vi "Clear Received Replies.vi"(8 "error in (no error)":errorcluster, 11 "Tamer in":refnum<class "Tamer.lvclass">) -> (0 "error out":errorcluster, 3 "Tamer out":refnum<class "Tamer.lvclass">)   [LabVIEW 2020, in "Tamer.lvlib" / "Tamer.lvclass"]
doc: "Clears lists of already received replies"
uses:
  Tamer.lvclass
  Reply.ctl
  Tamer.lvclass/Tamer.ctl
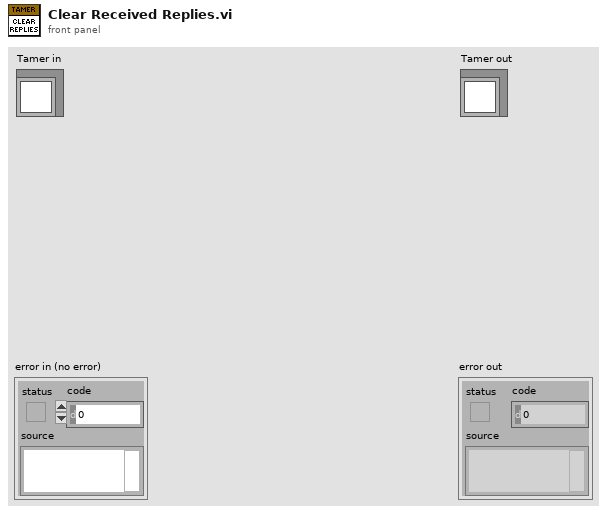
[diagram p1: front panel]
types:
  T1 = typedef "Tamer.lvlib/Tamer.lvclass/Reply.ctl" = cluster{"ID":string, "Status":bool, "GUID":string}
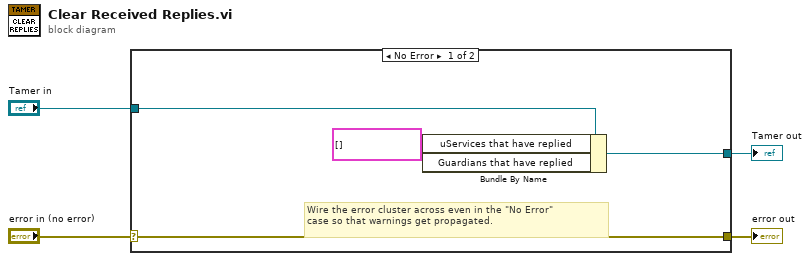
[diagram p0: block diagram]
diagram:
  n1 = case shown="No Error" "error in (no error)" {
    selector: "error in (no error)" -> [w8 w10]
    tunnel: [w8 w10] -> w3
    tunnel: [w6 w9] -> w1
    tunnel: "Tamer in" -> [w7 w9]
    frame No Error {
      w5 = T1[] [] ("uServices that have replied")
      # "Wire the error cluster across even in the \"No Error\"\ncase so that warnings get propagated."
      n2 = Bundle By Name(cluster=w7, "uServices that have replied"=w5, "Guardians that have replied"=w5) -> (w6:refnum<class "Tamer.lvclass">)
    }
    frame Error {
    }
  }
  "error out" <- w3
  "Tamer out" <- w1
